vi "BASE-Main.vi"() -> ()   [LabVIEW 2017]
uses:
  <vilib>/Utility/error.llb/DialogType.ctl
  55ed0eea-cd20-493f-8468-85b8c1a0a0c0.vi
panel:
  in  "PARAMETERS":bool
  in  "INPUT OUTPUT":bool
  in  "SETTING":bool
  in  "MANUAL":bool
  in  "RECIPE":bool
  out "error out":errorcluster
  in  "Logout":bool
  in  "Stop":bool
  in  "Create Login":bool
  in  "Reports":bool
  in  "Start":bool
  out "Time":string
  out "Date":string
  in  "Login":bool
  # "AUTO MOF"
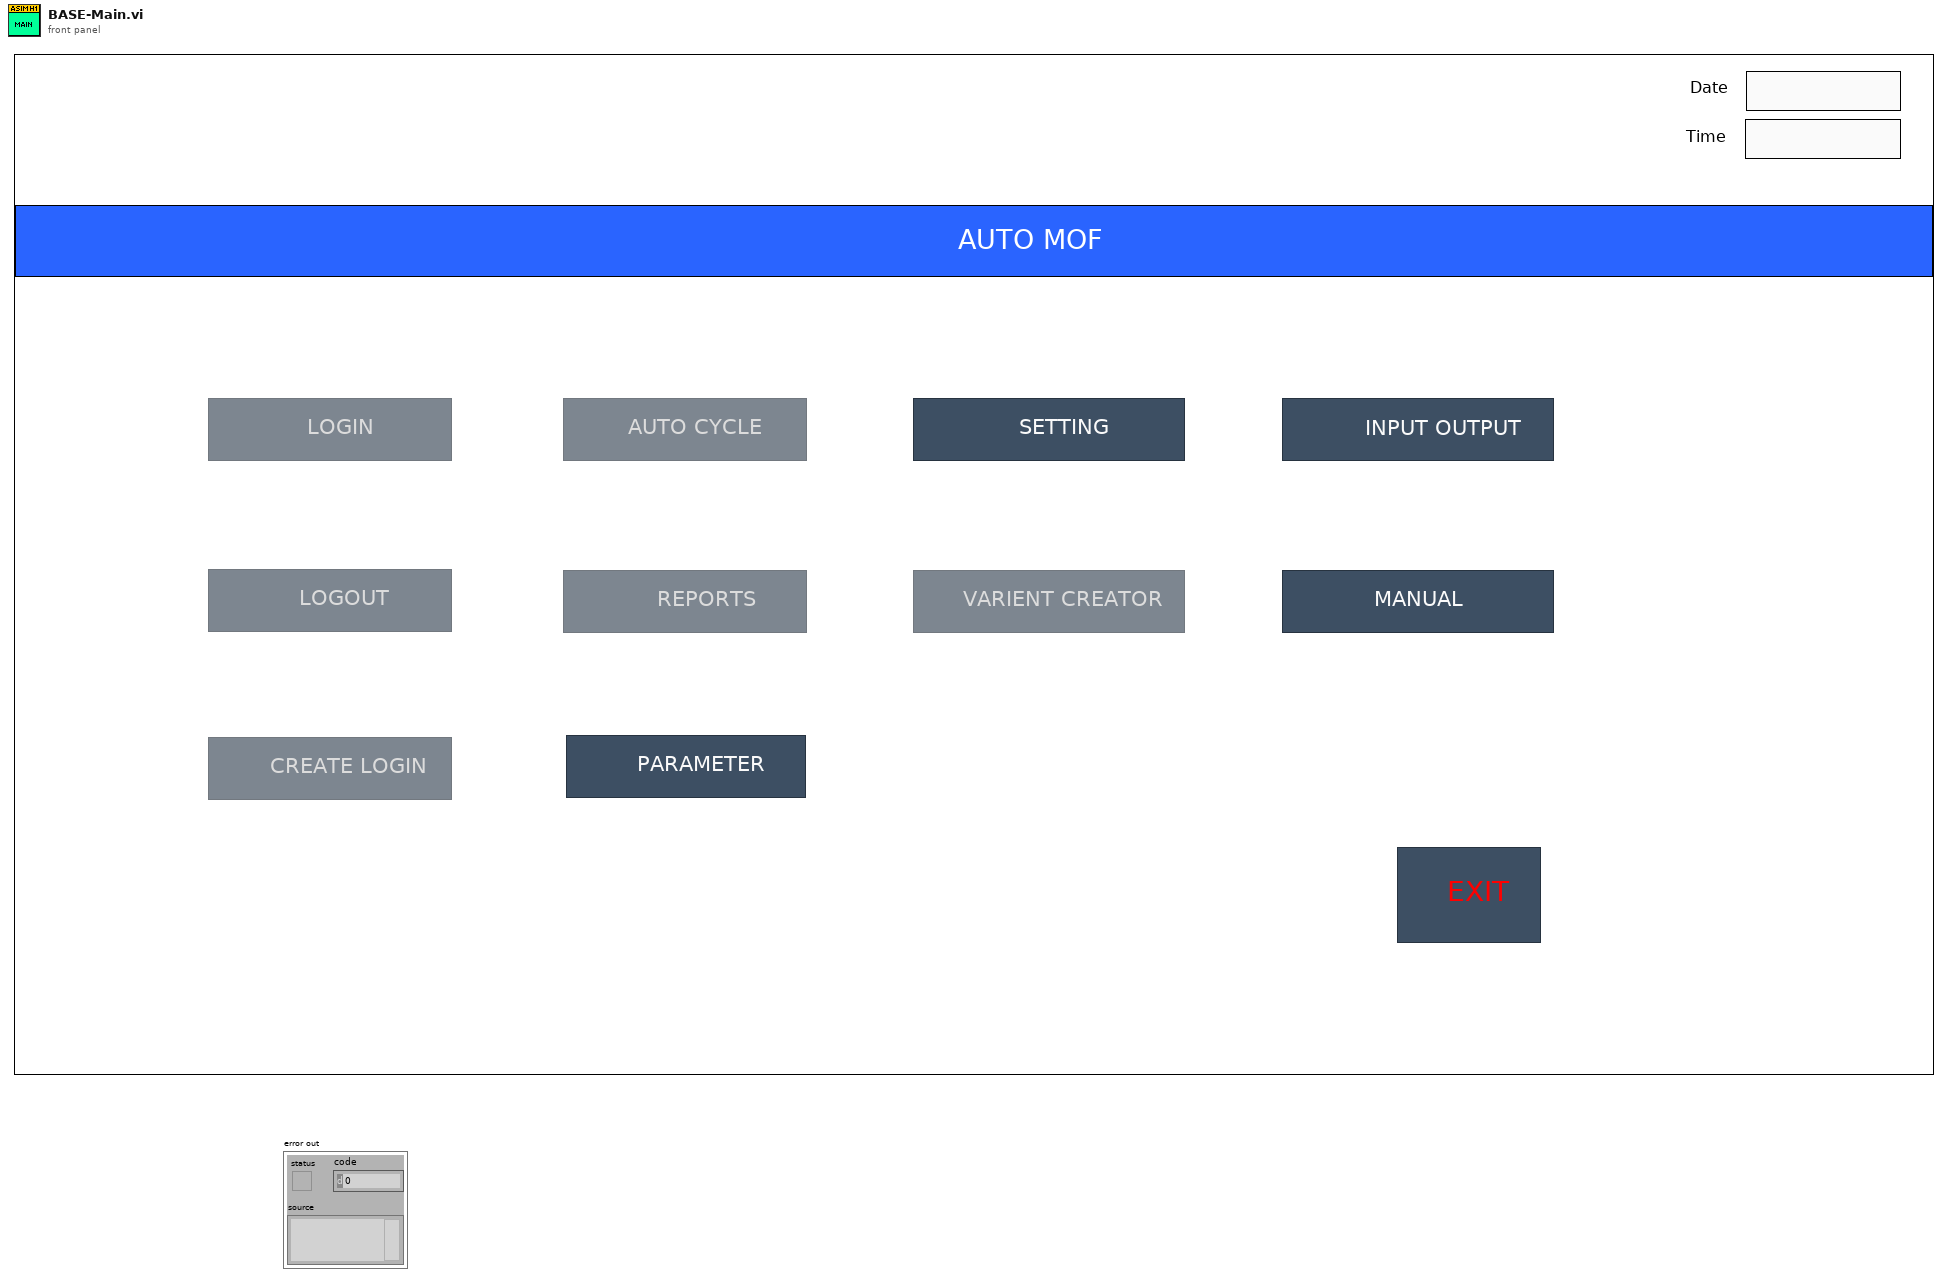
[diagram p1: front panel]
types:
  T1 = enum8{"Enabled", "Disabled", "Disabled and Grayed Out"}
  T2 = enum32{"Invalid", "Standard", "Closed", "Hidden", "Minimized", "Maximized"}
  T3 = typedef "DialogType.ctl" = u16
  T4 = enum32{"invalid app kind", "Development System", "Run Time System", "Student Edition", "Embedded LabVIEW", "Evaluation", "Custom"}
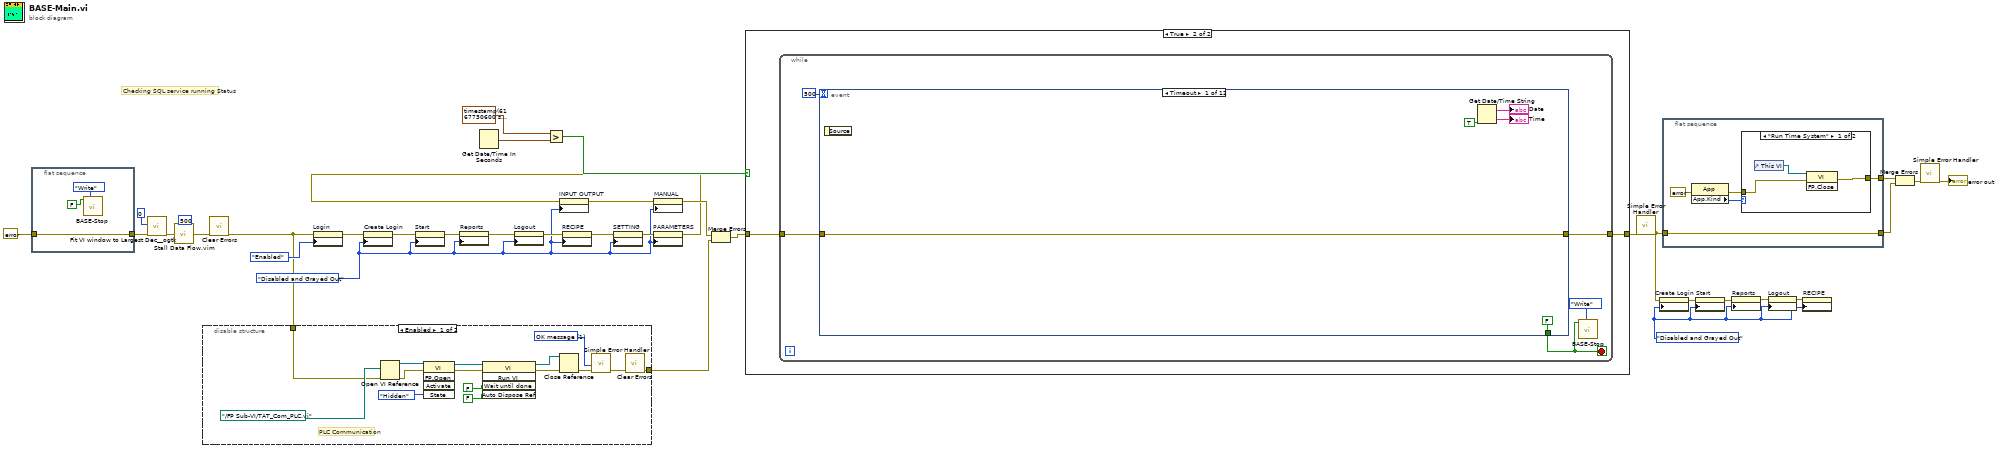
[diagram p0: block diagram]
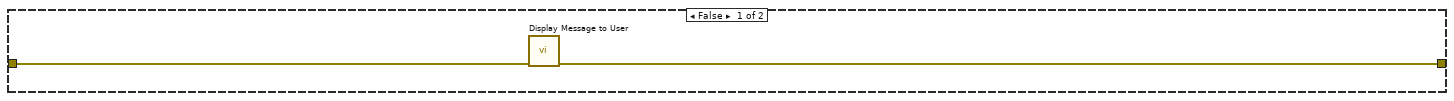
[diagram p4: hidden frame]
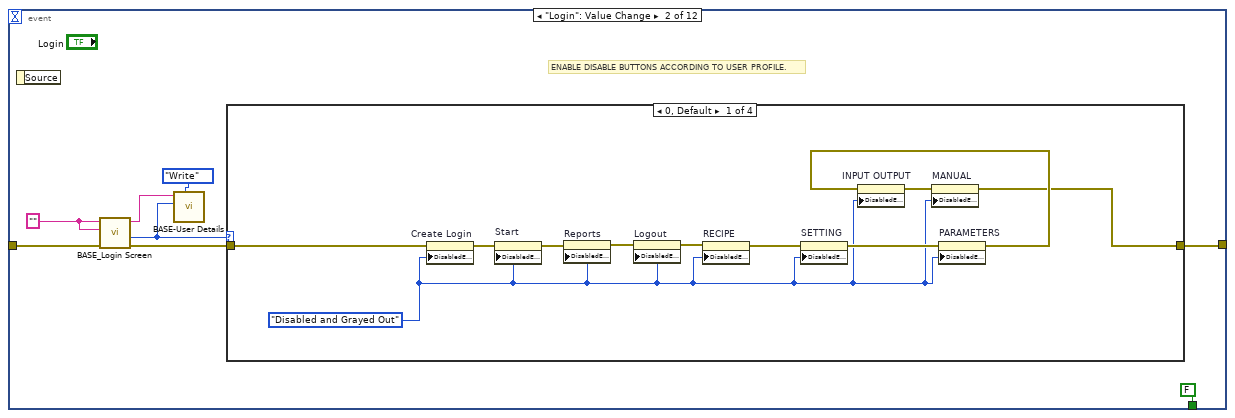
[diagram p5: hidden frame]
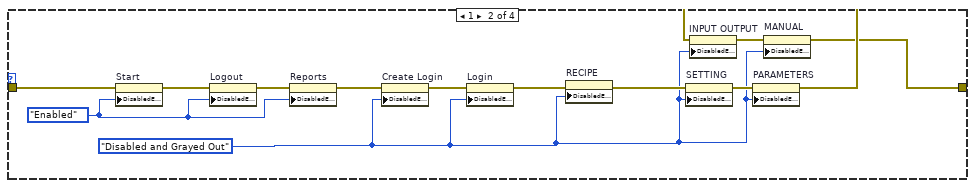
[diagram p6: hidden frame]
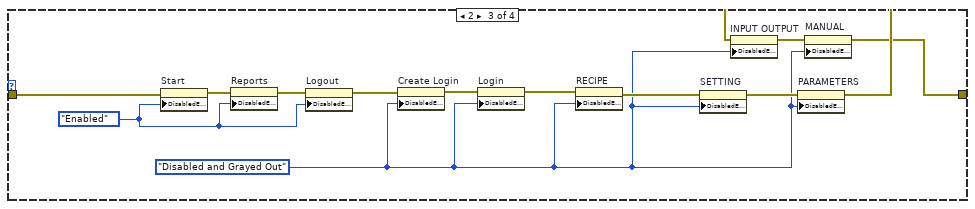
[diagram p7: hidden frame]
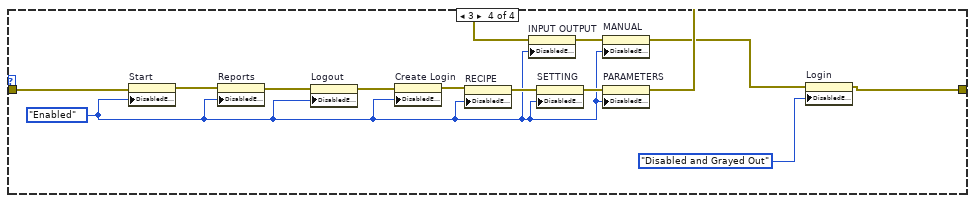
[diagram p8: hidden frame]
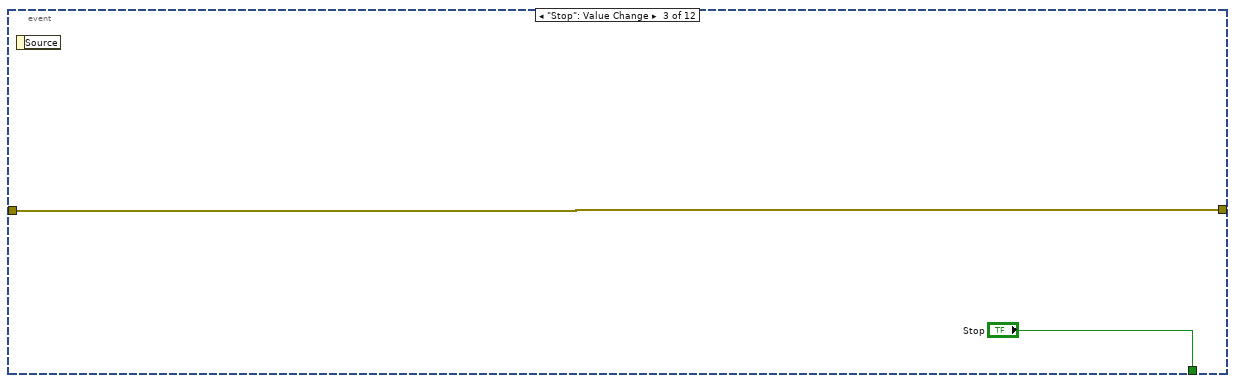
[diagram p9: hidden frame]
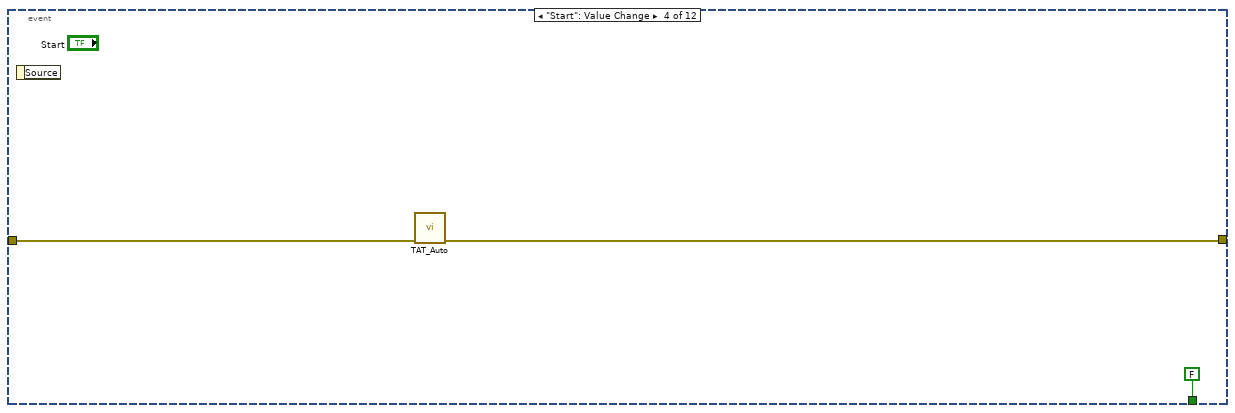
[diagram p10: hidden frame]
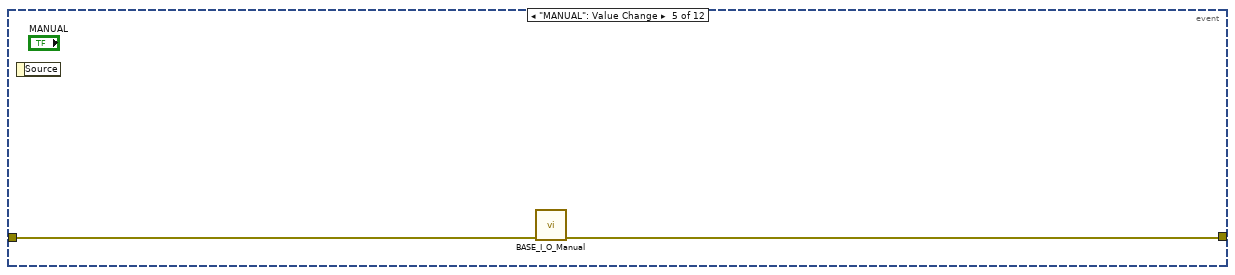
[diagram p11: hidden frame]
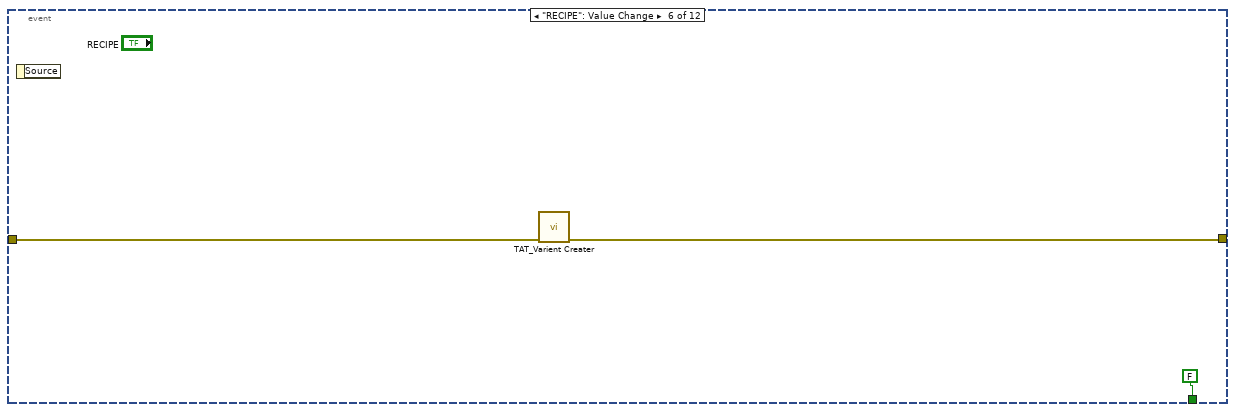
[diagram p12: hidden frame]
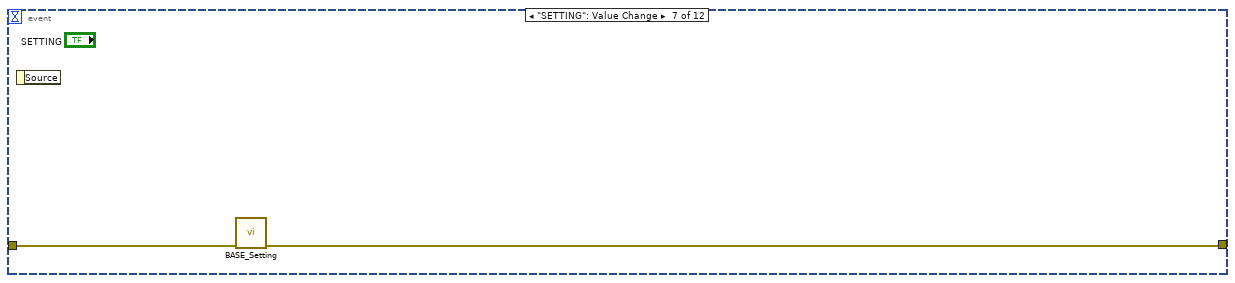
[diagram p13: hidden frame]
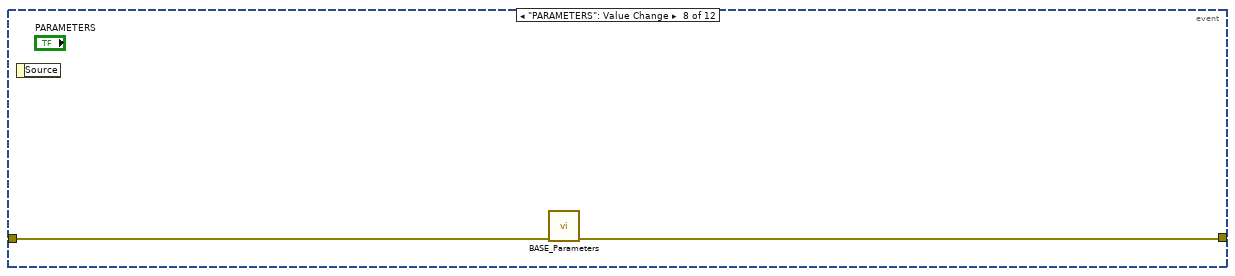
[diagram p14: hidden frame]
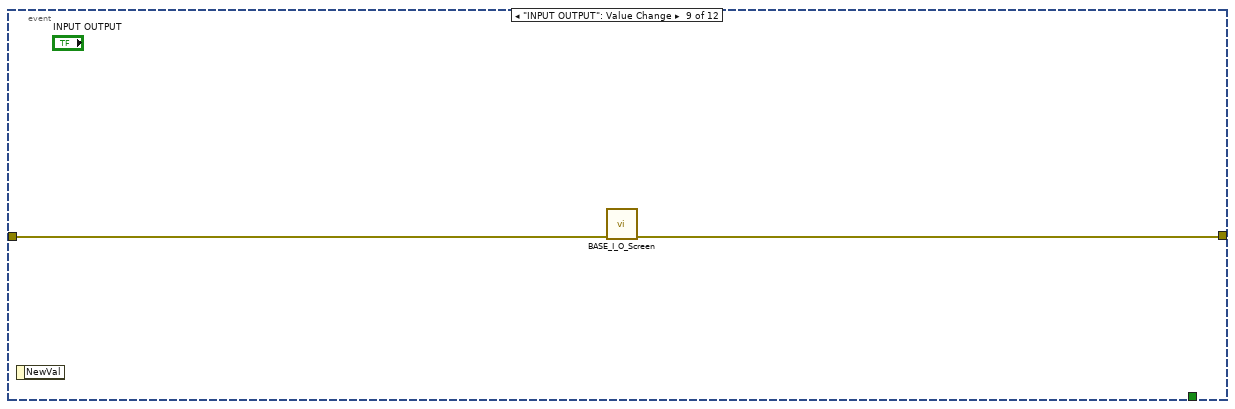
[diagram p15: hidden frame]
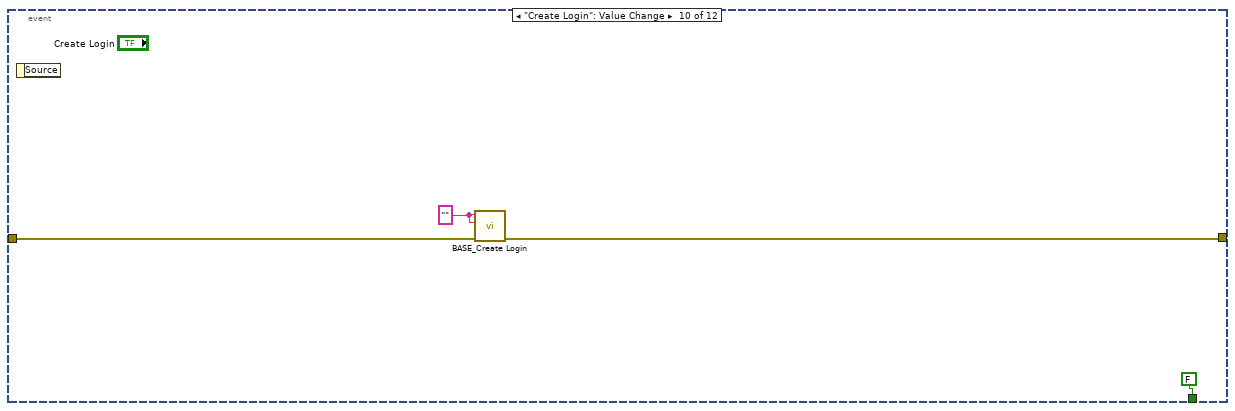
[diagram p16: hidden frame]
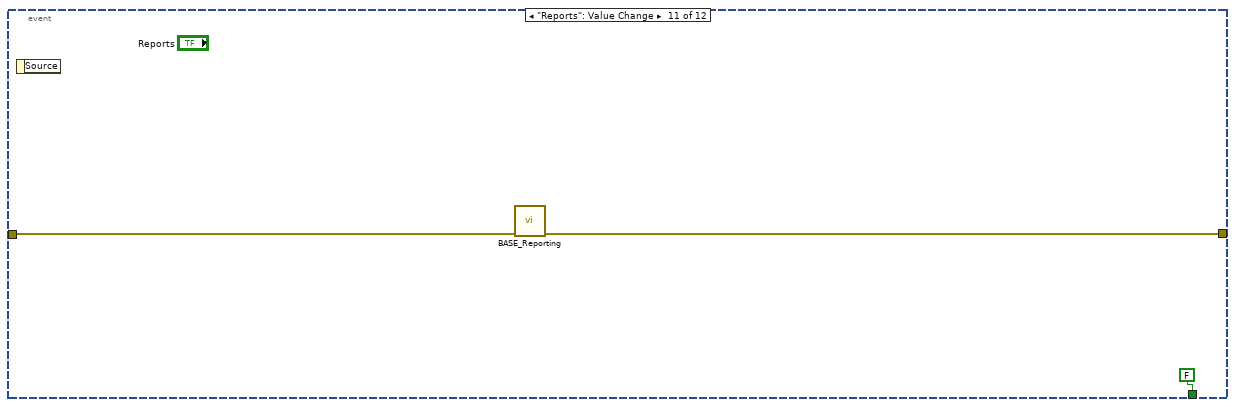
[diagram p17: hidden frame]
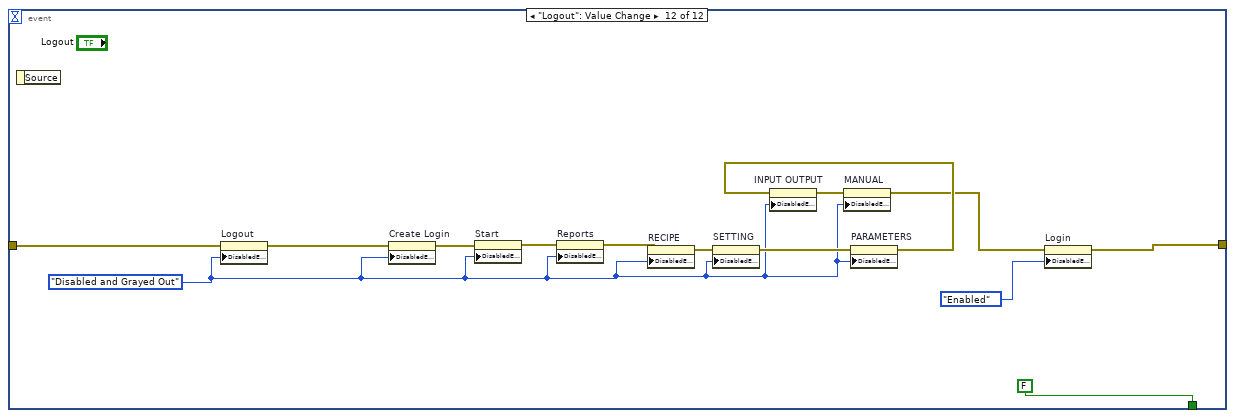
[diagram p18: hidden frame]
diagram:
  w13 = T1."Disabled and Grayed Out" ("Disabled")
  w1 = T1."Disabled and Grayed Out" ("Disabled")
  # "Checking SQL service running Status"
  n1 = flat-sequence {
    tunnel: [w38] -> w26
    tunnel: errorcluster {"status"=FALSE, "code"=0, "source"=""} ("error constant") -> [w38]
    frame #0 {
      n2 = call "BASE-Stop.vi"("Enum"=enum16{"Read", "Write"}."Write", "Stop"=FALSE) -> ()  [unwired: 9 in, 1 out]
    }
  }
  n3 = call <userlib>:"Fit VI window to Largest Dec__ogtk.vi"("error in (no error)"=w26, "border spacing (2 px)"=0) -> ("error out"=w18:errorcluster)  [unwired: 4 in, 1 out]
  n4 = call "Stall Data Flow.vim"("value in"=w18, "milliseconds to wait"=u32 500) -> ("value out"=w17:errorcluster)  [unwired: 1 out]
  n5 = call <vilib>:"Clear Errors.vi"("error in (no error)"=w17) -> ("error out"=w22:errorcluster)  [unwired: 5 in, 1 out]
  n6 = disable-structure shown="Enabled" {
    disable-tunnel: [w40 _] -> w24
    disable-tunnel: w22 -> [w39 _]
    frame Enabled {
      w42 = T3 1 items=["no dialog", "OK message", "continue or stop message", "OK message + warnings", "continue/stop + warnings"] ("type of dialog (OK msg:1)")
      # "PLC Communication"
      n7 = Open VI Reference(vi path=path "../FP Sub-VI/TAT_Com_PLC.vi", error in (no error)=w39) -> (vi reference=w50:refnum<vi>, error out=w51:errorcluster)  [unwired: 4 in]
      n8 = invoke class="VI" method="FP.Open"(reference=w50, error in=w51, "State"=T2."Hidden") -> (reference out=w53:refnum<vi>, error out=w52:errorcluster)  [unwired: 2 in, 3 out]
      n9 = invoke class="VI" method="Run VI"(reference=w53, error in=w52, "Wait until done"=FALSE ("Wait Until Done"), "Auto Dispose Ref"=FALSE ("Auto Dispose Reference")) -> (reference out=w49:refnum<vi>, error out=w48:errorcluster)  [unwired: 1 in, 3 out]
      n10 = Close Reference(reference=w49, error in (no error)=w48) -> (error out=w43:errorcluster)
      n11 = call <vilib>:"Simple Error Handler.vi"("type of dialog (OK msg:1)"=w42, "error in (no error)"=w43) -> ("error out"=w41:errorcluster)  [unwired: 3 in, 4 out]
      n12 = call <vilib>:"Clear Errors.vi"("error in (no error)"=w41) -> ("error out"=w40:errorcluster)  [unwired: 5 in, 1 out]
    }
    frame Disabled {
    }
  }
  n13 = property on="Login" class="Bool"(error in=w22, "DisabledEnum"=T1."Enabled" ("Disabled")) -> (error out=w30:errorcluster)  [unwired: 1 in, 1 out]
  n14 = property on="Create Login" class="Bool"(error in=w30, "DisabledEnum"=w1) -> (error out=w34:errorcluster)  [unwired: 1 in, 1 out]
  n15 = property on="Start" class="Bool"(error in=w34, "DisabledEnum"=w1) -> (error out=w14:errorcluster)  [unwired: 1 in, 1 out]
  n16 = property on="Reports" class="Bool"(error in=w14, "DisabledEnum"=w1) -> (error out=w28:errorcluster)  [unwired: 1 in, 1 out]
  n17 = Get Date/Time In Seconds() -> (seconds since 1Jan1904=w20:timestamp)
  n18 = property on="Logout" class="Bool"(error in=w28, "DisabledEnum"=w1) -> (error out=w15:errorcluster)  [unwired: 1 in, 1 out]
  n19 = Greater?(x=timestamp(6167730600 s since 1904-01-01), y=w20) -> (0:w19:bool)
  n20 = property on="RECIPE" class="Bool"(error in=w15, "DisabledEnum"=w1) -> (error out=w7:errorcluster)  [unwired: 1 in, 1 out]
  n21 = property on="SETTING" class="Bool"(error in=w7, "DisabledEnum"=w1) -> (error out=w5:errorcluster)  [unwired: 1 in, 1 out]
  n22 = property on="PARAMETERS" class="Bool"(error in=w5, "DisabledEnum"=w1) -> (error out=w2:errorcluster)  [unwired: 1 in, 1 out]
  n23 = property on="INPUT OUTPUT" class="Bool"(error in=w2, "DisabledEnum"=w1) -> (error out=w3:errorcluster)  [unwired: 1 in, 1 out]
  n24 = property on="MANUAL" class="Bool"(error in=w3, "DisabledEnum"=w1) -> (error out=w4:errorcluster)  [unwired: 1 in, 1 out]
  n25 = Merge Errors(w4, w24) -> (w25:errorcluster)
  n26 = case shown="True" w19 {
    tunnel: w25 -> [w55 w57]
    tunnel: [w54 w56] -> w35
    frame False {
      n27 = call "Display Message to User"("error in (no error)"=w55) -> ("error out"=w54:errorcluster)  [unwired: 9 in, 1 out]
    }
    frame True {
      n28 = while {
        tunnel: w57 -> [w61]
        tunnel: [w60] -> w56
        stop <- w58 stop-if-true
        n29 = event shown="[0] Timeout" {
          selector: _ -> [_ _ _ _ _ _ _ _ _ _ _ _]
          dyn-events: _ -> [_ _ _ _ _ _ _ _ _ _ _ _]
          timeout: 500 -> [_ _ _ _ _ _ _ _ _ _ _ _]
          tunnel: w61 -> [w65 w75 w126 w129 w132 w134 w137 w139 w141 w145 w147 w159]
          tunnel: [w65 w68 w126 w128 w131 w133 w136 w138 w140 w144 w146 w160] -> w60
          tunnel: [FALSE ("Stop") FALSE ("Stop") "Stop" FALSE ("Stop") _ FALSE ("Stop") _ _ _ FALSE ("Stop") FALSE ("Stop") FALSE ("Stop")] -> w58
          event Timeout {
            n30 = event-data() -> ()  [unwired: 1 in, 1 out]
            n31 = Get Date/Time String(want seconds? (F)=TRUE) -> (date string=→"Date":string, time string=→"Time":string)  [unwired: 2 in]
          }
          event "Login": Value Change {
            w71 = "" ("User Name")
            # "ENABLE DISABLE BUTTONS ACCORDING TO USER PROFILE."
            n32 = event-data() -> ()  [unwired: 1 in, 1 out]
            n33 = call "BASE_Login Screen.vi"("Error In"=w75, "Password"=w71, "User Name"=w71) -> ("error out"=w74:errorcluster, "Level"=w69:i32, "User Name Out"=w72:string)  [unwired: 5 in, 1 out]
            n34 = call "BASE-User Details.vi"("Enum"=enum16{"Read", "Write"}."Write", "Level In"=w69, "User Name In"=w72) -> ()  [unwired: 7 in, 2 out]
            n35 = case shown="0, Default" w69 {
              tunnel: w74 -> [w84 w99 w112 w125]
              tunnel: [w77 w87 w101 w119] -> w68
              frame 0, Default {
                w76 = T1."Disabled and Grayed Out" ("Disabled")
                n36 = property on="Create Login" class="Bool"(error in=w84, "DisabledEnum"=w76) -> (error out=w86:errorcluster)  [unwired: 1 in, 1 out]
                n37 = property on="Start" class="Bool"(error in=w86, "DisabledEnum"=w76) -> (error out=w85:errorcluster)  [unwired: 1 in, 1 out]
                n38 = property on="Reports" class="Bool"(error in=w85, "DisabledEnum"=w76) -> (error out=w82:errorcluster)  [unwired: 1 in, 1 out]
                n39 = property on="Logout" class="Bool"(error in=w82, "DisabledEnum"=w76) -> (error out=w83:errorcluster)  [unwired: 1 in, 1 out]
                n40 = property on="RECIPE" class="Bool"(error in=w83, "DisabledEnum"=w76) -> (error out=w81:errorcluster)  [unwired: 1 in, 1 out]
                n41 = property on="SETTING" class="Bool"(error in=w81, "DisabledEnum"=w76) -> (error out=w80:errorcluster)  [unwired: 1 in, 1 out]
                n42 = property on="PARAMETERS" class="Bool"(error in=w80, "DisabledEnum"=w76) -> (error out=w79:errorcluster)  [unwired: 1 in, 1 out]
                n43 = property on="INPUT OUTPUT" class="Bool"(error in=w79, "DisabledEnum"=w76) -> (error out=w78:errorcluster)  [unwired: 1 in, 1 out]
                n44 = property on="MANUAL" class="Bool"(error in=w78, "DisabledEnum"=w76) -> (error out=w77:errorcluster)  [unwired: 1 in, 1 out]
              }
              frame 1 {
                w88 = T1."Disabled and Grayed Out" ("Disabled")
                w93 = T1."Enabled" ("Disabled")
                n45 = property on="Start" class="Bool"(error in=w99, "DisabledEnum"=w93) -> (error out=w95:errorcluster)  [unwired: 1 in, 1 out]
                n46 = property on="Logout" class="Bool"(error in=w95, "DisabledEnum"=w93) -> (error out=w97:errorcluster)  [unwired: 1 in, 1 out]
                n47 = property on="Reports" class="Bool"(error in=w97, "DisabledEnum"=w93) -> (error out=w98:errorcluster)  [unwired: 1 in, 1 out]
                n48 = property on="Create Login" class="Bool"(error in=w98, "DisabledEnum"=w88) -> (error out=w96:errorcluster)  [unwired: 1 in, 1 out]
                n49 = property on="Login" class="Bool"(error in=w96, "DisabledEnum"=w88) -> (error out=w94:errorcluster)  [unwired: 1 in, 1 out]
                n50 = property on="RECIPE" class="Bool"(error in=w94, "DisabledEnum"=w88) -> (error out=w92:errorcluster)  [unwired: 1 in, 1 out]
                n51 = property on="SETTING" class="Bool"(error in=w92, "DisabledEnum"=w88) -> (error out=w91:errorcluster)  [unwired: 1 in, 1 out]
                n52 = property on="PARAMETERS" class="Bool"(error in=w91, "DisabledEnum"=w88) -> (error out=w89:errorcluster)  [unwired: 1 in, 1 out]
                n53 = property on="INPUT OUTPUT" class="Bool"(error in=w89, "DisabledEnum"=w88) -> (error out=w90:errorcluster)  [unwired: 1 in, 1 out]
                n54 = property on="MANUAL" class="Bool"(error in=w90, "DisabledEnum"=w88) -> (error out=w87:errorcluster)  [unwired: 1 in, 1 out]
              }
              frame 2 {
                w100 = T1."Disabled and Grayed Out" ("Disabled")
                w106 = T1."Enabled" ("Disabled")
                n55 = property on="Start" class="Bool"(error in=w112, "DisabledEnum"=w106) -> (error out=w109:errorcluster)  [unwired: 1 in, 1 out]
                n56 = property on="Reports" class="Bool"(error in=w109, "DisabledEnum"=w106) -> (error out=w111:errorcluster)  [unwired: 1 in, 1 out]
                n57 = property on="Logout" class="Bool"(error in=w111, "DisabledEnum"=w106) -> (error out=w107:errorcluster)  [unwired: 1 in, 1 out]
                n58 = property on="Create Login" class="Bool"(error in=w107, "DisabledEnum"=w100) -> (error out=w110:errorcluster)  [unwired: 1 in, 1 out]
                n59 = property on="Login" class="Bool"(error in=w110, "DisabledEnum"=w100) -> (error out=w108:errorcluster)  [unwired: 1 in, 1 out]
                n60 = property on="RECIPE" class="Bool"(error in=w108, "DisabledEnum"=w100) -> (error out=w105:errorcluster)  [unwired: 1 in, 1 out]
                n61 = property on="SETTING" class="Bool"(error in=w105, "DisabledEnum"=w100) -> (error out=w104:errorcluster)  [unwired: 1 in, 1 out]
                n62 = property on="PARAMETERS" class="Bool"(error in=w104, "DisabledEnum"=w100) -> (error out=w102:errorcluster)  [unwired: 1 in, 1 out]
                n63 = property on="INPUT OUTPUT" class="Bool"(error in=w102, "DisabledEnum"=w100) -> (error out=w103:errorcluster)  [unwired: 1 in, 1 out]
                n64 = property on="MANUAL" class="Bool"(error in=w103, "DisabledEnum"=w100) -> (error out=w101:errorcluster)  [unwired: 1 in, 1 out]
              }
              frame 3 {
                w114 = T1."Enabled" ("Disabled")
                n65 = property on="Start" class="Bool"(error in=w125, "DisabledEnum"=w114) -> (error out=w121:errorcluster)  [unwired: 1 in, 1 out]
                n66 = property on="Reports" class="Bool"(error in=w121, "DisabledEnum"=w114) -> (error out=w124:errorcluster)  [unwired: 1 in, 1 out]
                n67 = property on="Logout" class="Bool"(error in=w124, "DisabledEnum"=w114) -> (error out=w123:errorcluster)  [unwired: 1 in, 1 out]
                n68 = property on="Create Login" class="Bool"(error in=w123, "DisabledEnum"=w114) -> (error out=w122:errorcluster)  [unwired: 1 in, 1 out]
                n69 = property on="RECIPE" class="Bool"(error in=w122, "DisabledEnum"=w114) -> (error out=w118:errorcluster)  [unwired: 1 in, 1 out]
                n70 = property on="SETTING" class="Bool"(error in=w118, "DisabledEnum"=w114) -> (error out=w117:errorcluster)  [unwired: 1 in, 1 out]
                n71 = property on="PARAMETERS" class="Bool"(error in=w117, "DisabledEnum"=w114) -> (error out=w115:errorcluster)  [unwired: 1 in, 1 out]
                n72 = property on="INPUT OUTPUT" class="Bool"(error in=w115, "DisabledEnum"=w114) -> (error out=w116:errorcluster)  [unwired: 1 in, 1 out]
                n73 = property on="MANUAL" class="Bool"(error in=w116, "DisabledEnum"=w114) -> (error out=w113:errorcluster)  [unwired: 1 in, 1 out]
                n74 = property on="Login" class="Bool"(error in=w113, "DisabledEnum"=T1."Disabled and Grayed Out" ("Disabled")) -> (error out=w119:errorcluster)  [unwired: 1 in, 1 out]
              }
            }
          }
          event "Stop": Value Change {
            n75 = event-data() -> ()  [unwired: 1 in, 1 out]
          }
          event "Start": Value Change {
            n76 = event-data() -> ()  [unwired: 1 in, 1 out]
            n77 = call "TAT_Auto.vi"("error in (no error)"=w129) -> ("error out"=w128:errorcluster)  [unwired: 10 in]
          }
          event "MANUAL": Value Change {
            n78 = event-data() -> ()  [unwired: 1 in, 1 out]
            n79 = call "BASE_I_O_Manual.vi"("error in (no error)"=w132) -> ("error out"=w131:errorcluster)  [unwired: 10 in]
          }
          event "RECIPE": Value Change {
            n80 = event-data() -> ()  [unwired: 1 in, 1 out]
            n81 = call "TAT_Varient Creater.vi"("error in (no error)"=w134) -> ("error out"=w133:errorcluster)  [unwired: 10 in]
          }
          event "SETTING": Value Change {
            n82 = event-data() -> ()  [unwired: 1 in, 1 out]
            n83 = call "BASE_Setting.vi"("error in (no error)"=w137) -> ("error out"=w136:errorcluster)  [unwired: 10 in]
          }
          event "PARAMETERS": Value Change {
            n84 = event-data() -> ()  [unwired: 1 in, 1 out]
            n85 = call "BASE_Parameters.vi"("error in (no error)"=w139) -> ("error out"=w138:errorcluster)  [unwired: 10 in]
          }
          event "INPUT OUTPUT": Value Change {
            n86 = event-data() -> ()  [unwired: 1 in, 1 out]
            n87 = call "BASE_I_O_Screen.vi"("error in (no error)"=w141) -> ("error out"=w140:errorcluster)  [unwired: 10 in]
          }
          event "Create Login": Value Change {
            w143 = "" ("User Name")
            n88 = event-data() -> ()  [unwired: 1 in, 1 out]
            n89 = call "BASE_Create Login.vi"("Error In"=w145, "Password"=w143, "User Name"=w143) -> ("error out"=w144:errorcluster)  [unwired: 6 in]
          }
          event "Reports": Value Change {
            n90 = event-data() -> ()  [unwired: 1 in, 1 out]
            n91 = call "BASE_Reporting.vi"("error in (no error)"=w147) -> ("error out"=w146:errorcluster)  [unwired: 10 in]
          }
          event "Logout": Value Change {
            w149 = T1."Disabled and Grayed Out" ("Disabled")
            n92 = event-data() -> ()  [unwired: 1 in, 1 out]
            n93 = property on="Logout" class="Bool"(error in=w159, "DisabledEnum"=w149) -> (error out=w155:errorcluster)  [unwired: 1 in, 1 out]
            n94 = property on="Create Login" class="Bool"(error in=w155, "DisabledEnum"=w149) -> (error out=w162:errorcluster)  [unwired: 1 in, 1 out]
            n95 = property on="Start" class="Bool"(error in=w162, "DisabledEnum"=w149) -> (error out=w161:errorcluster)  [unwired: 1 in, 1 out]
            n96 = property on="Reports" class="Bool"(error in=w161, "DisabledEnum"=w149) -> (error out=w156:errorcluster)  [unwired: 1 in, 1 out]
            n97 = property on="RECIPE" class="Bool"(error in=w156, "DisabledEnum"=w149) -> (error out=w152:errorcluster)  [unwired: 1 in, 1 out]
            n98 = property on="SETTING" class="Bool"(error in=w152, "DisabledEnum"=w149) -> (error out=w154:errorcluster)  [unwired: 1 in, 1 out]
            n99 = property on="PARAMETERS" class="Bool"(error in=w154, "DisabledEnum"=w149) -> (error out=w151:errorcluster)  [unwired: 1 in, 1 out]
            n100 = property on="INPUT OUTPUT" class="Bool"(error in=w151, "DisabledEnum"=w149) -> (error out=w153:errorcluster)  [unwired: 1 in, 1 out]
            n101 = property on="MANUAL" class="Bool"(error in=w153, "DisabledEnum"=w149) -> (error out=w150:errorcluster)  [unwired: 1 in, 1 out]
            n102 = property on="Login" class="Bool"(error in=w150, "DisabledEnum"=T1."Enabled" ("Disabled")) -> (error out=w160:errorcluster)  [unwired: 1 in, 1 out]
          }
        }
        n103 = call "BASE-Stop.vi"("Enum"=enum16{"Read", "Write"}."Write", "Stop"=w58) -> ()  [unwired: 9 in, 1 out]
      }
    }
  }
  n104 = call <vilib>:"Simple Error Handler.vi"("error in (no error)"=w35) -> ("error out"=w8:errorcluster)  [unwired: 4 in, 4 out]
  n105 = property on="Create Login" class="Bool"(error in=w8, "DisabledEnum"=w13) -> (error out=w9:errorcluster)  [unwired: 1 in, 1 out]
  n106 = flat-sequence {
    tunnel: [w164] -> w33
    tunnel: [w163] -> w31
    tunnel: w8 -> [w163]
    frame #0 {
      n107 = property class="App"(error in=errorcluster {"status"=FALSE, "code"=0, "source"=""} ("error in (no error)")) -> (error out=w166:errorcluster, "App.Kind"=w167:T4)  [unwired: 1 in, 1 out]
      n108 = case shown="\"Run Time System\"" w167 {
        tunnel: w166 -> [w169 w171]
        tunnel: [w168 w171] -> w164
        frame "Run Time System" {
          n109 = control-ref of="This VI"() -> (w170:refnum<vi>)
          n110 = invoke class="VI" method="FP.Close"(reference=w170, error in=w169) -> (error out=w168:errorcluster)  [unwired: 1 in, 2 out]
        }
        frame "Development System", Default {
        }
      }
    }
  }
  n111 = property on="Start" class="Bool"(error in=w9, "DisabledEnum"=w13) -> (error out=w12:errorcluster)  [unwired: 1 in, 1 out]
  n112 = property on="Reports" class="Bool"(error in=w12, "DisabledEnum"=w13) -> (error out=w10:errorcluster)  [unwired: 1 in, 1 out]
  n113 = property on="Logout" class="Bool"(error in=w10, "DisabledEnum"=w13) -> (error out=w11:errorcluster)  [unwired: 1 in, 1 out]
  n114 = property on="RECIPE" class="Bool"(error in=w11, "DisabledEnum"=w13) -> ()  [unwired: 1 in, 2 out]
  n115 = Merge Errors(w33, w31) -> (w32:errorcluster)
  n116 = call <vilib>:"Simple Error Handler.vi"("error in (no error)"=w32) -> ("error out"=→"error out":errorcluster)  [unwired: 4 in, 4 out]
